vi "Test Indicator.vi"() -> ()   [LabVIEW 2020, in "VolatusGUIElements.lvlib" / "GaugeIndicator.lvclass"]
uses:
  GaugeIndicator.lvclass
  C:/dev/lv20CE/relink/lv-volatus/VolatusGUI/GUI Element/GUI Element.lvclass
  Volatus/VolatusAPI/VolatusAPI.lvclass
  GaugeIndicator.lvclass/GaugeIndicator.ctl
  VolatusGUI/GUI Element/GUI Element.lvclass
panel:
  out "GUI Element out":refnum<class "GaugeIndicator.lvclass">
  out "error out":errorcluster
  out "GaugeIndicator":T1={"Color Band"=bytes[168], "Gauge"=1600.0, "High"=2500.0, "Low"=0.0} {"Gauge" scale=0.0..2500.0}
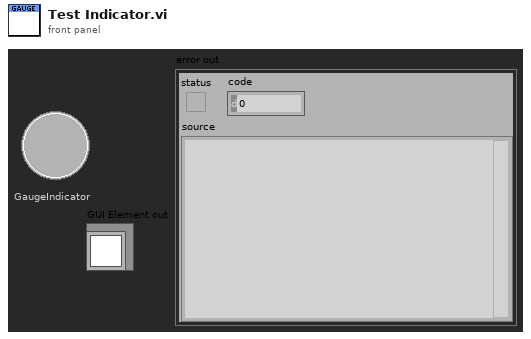
[diagram p1: front panel]
types:
  T1 = cluster{"Color Band":picture, "Gauge":dbl, "High":dbl, "Low":dbl}
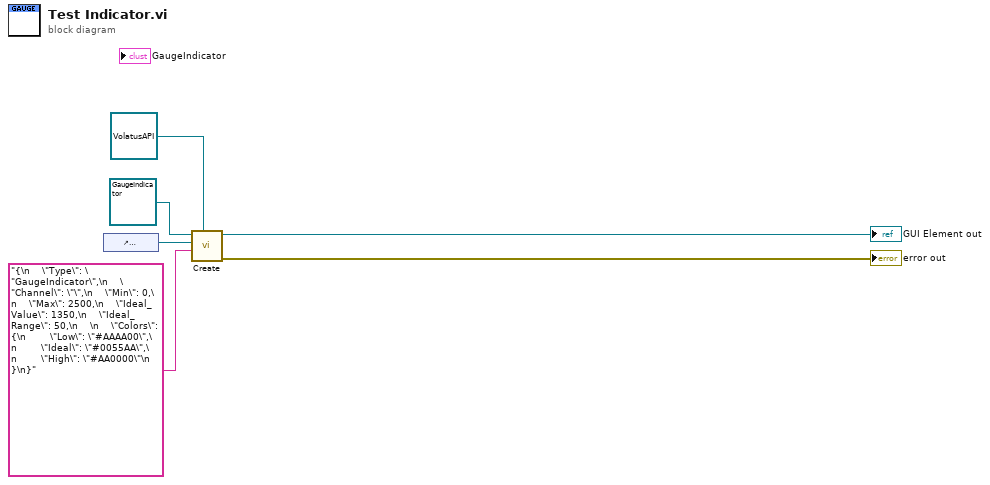
[diagram p0: block diagram]
diagram:
  n1 = control-ref of="GaugeIndicator"() -> (w6:refnum<vi>)
  n2 = call "Create.vi"("VolatusAPI"=refnum<class "VolatusAPI.lvclass"> refnum, "JSON"="{\n    \"Type\": \"GaugeIndicator\",\n    \"Channel\": \"\",\n    \"Min\": 0,\n    \"Max\": 2500,\n    \"Ideal_Value\": 1350,\n    \"Ideal_Range\": 50,\n    \n    \"Colors\": {\n        \"Low\": \"#AAAA00\",\n        \"Ideal\": \"#0055AA\",\n        \"High\": \"#AA0000\"\n    }\n}", "Ref"=w6, "GUI Element in"=refnum<class "GaugeIndicator.lvclass"> refnum ("VolatusGUIElements.lvlib:GaugeIndicator.lvclass")) -> ("error out"=→"error out":errorcluster, "GUI Element out"=→"GUI Element out":refnum<class "GaugeIndicator.lvclass">)  [unwired: 6 in]
